vi "CANOpen Enter Frame Information.vi"(5 "Type":T3=enum."TPDO", 7 "Edit?":bool, 8 "error in (no error)":errorcluster, 9 "PDO Channel":u8(ring) items=["PDO 1", "PDO 2", "PDO 3", "PDO 4"], 10 "Parameters":T5[](array[typedef]) {"Bit Offset" max=8 step=1; "Byte Offset" max=8 step=1}, 11 "Node Ptr":u64 format="%.0x") -> (0 "error out":errorcluster, 1 "Cancelled?":bool, 2 "PDO Settings":T4={"Parameters"=[], "PDO Channel"=1, "Start Index"=1, "Length"=0} {"PDO Channel" items=["PDO 1", "PDO 2", "PDO 3", "PDO 4"]; "Parameters"."Bit Offset" max=8 step=1; "Parameters"."Byte Offset" max=8 step=1}, 3 "Item Ref out":T8 format="%.0x")   [LabVIEW 2021, in "CANOpen Addon System Explorer.lvlib"]
uses:
  CANOpen Addon System Explorer.lvlib
  <vilib>/NI VeriStand/Custom Device API/Custom Device Item Ref.ctl
  Shared/CANOpen_PDO Parameter Settings.ctl
  Shared/CANOpen_PDO Data Type.ctl
  CANopen Byte Order.ctl
  Shared/CANOpen_PDO Settings.ctl
  CANOpen_PDO Type.ctl
  Import.ctl
  Export.ctl
  <vilib>/NI VeriStand/Custom Device API/Custom Device API.lvlib
  Shared/CANOpen Addon Shared.lvlib
panel:
  in  "Import":T1
  in  "Export":T2
  in  "Cancel Button":bool
  in  "OK Button":bool
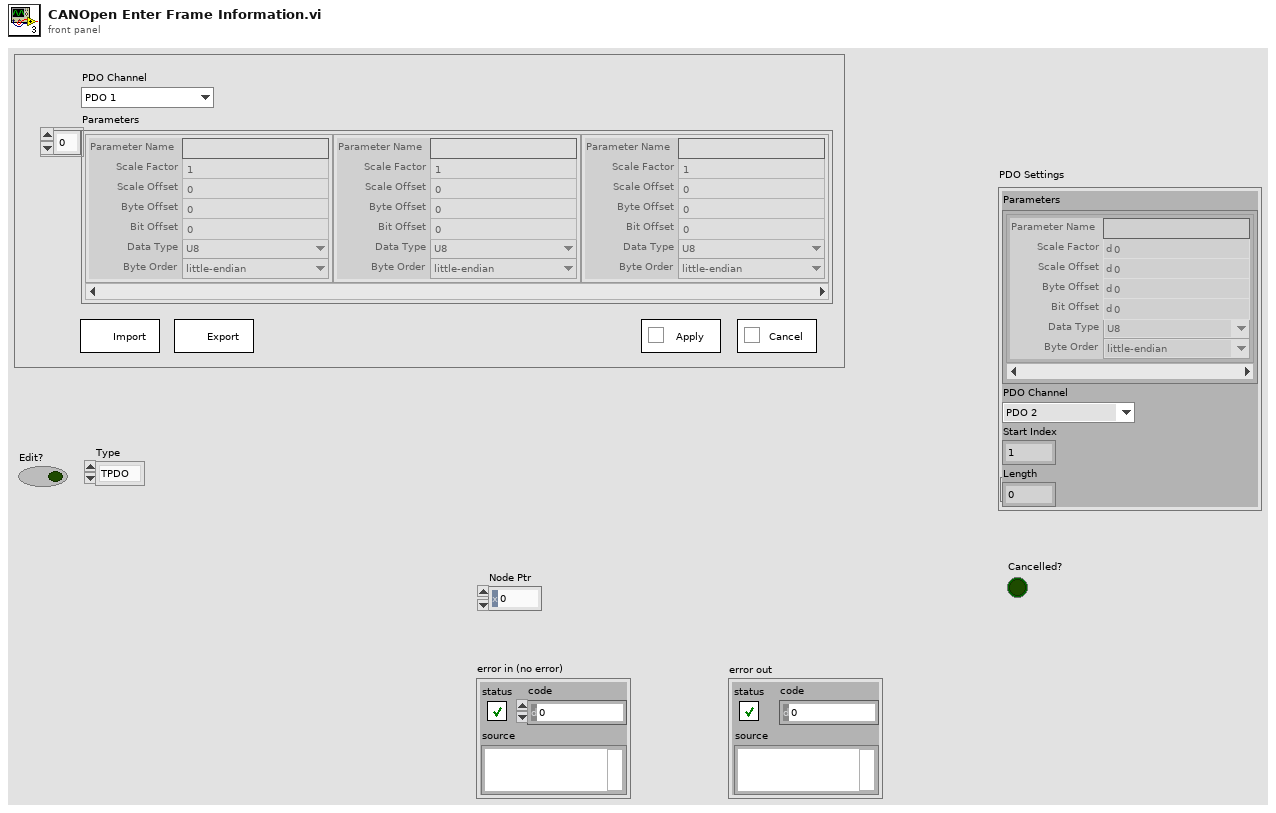
[diagram p1: front panel]
types:
  T1 = typedef "CANOpen Addon System Explorer.lvlib/Import.ctl" = bool
  T2 = typedef "CANOpen Addon System Explorer.lvlib/Export.ctl" = bool
  T3 = typedef "CANOpen Addon System Explorer.lvlib/CANOpen_PDO Type.ctl" = enum16{"RPDO", "TPDO"}
  T4 = typedef "CANOpen Addon Shared.lvlib/CANOpen_PDO Settings.ctl" = cluster{"Parameters":T5[], "PDO Channel":u8, "Start Index":u32, "Length":u32}
  T5 = typedef "CANOpen Addon Shared.lvlib/CANOpen_PDO Parameter Settings.ctl" = cluster{"Parameter Name":string, "Scale Factor":dbl, "Scale Offset":dbl, "Byte Offset":u8, "Bit Offset":u8, "Data Type":T6, "Byte Order":T7}
  T6 = typedef "CANOpen Addon Shared.lvlib/CANOpen_PDO Data Type.ctl" = enum16{"U8", "U16", "U32", "I8", "I16", "I32", "Single", "Double", "Boolean"}
  T7 = typedef "CANOpen Addon System Explorer.lvlib/CANopen Byte Order.ctl" = enum16{"big-endian network order", "little-endian"}
  T8 = typedef "Custom Device API.lvlib/Custom Device Item Ref.ctl" = u64
  T9 = typedef "Custom Device API.lvlib/Custom Device Item Info.ctl" = cluster{"Name":string, "Is Channel":bool, "GUID":string, "Is Waveform":bool}
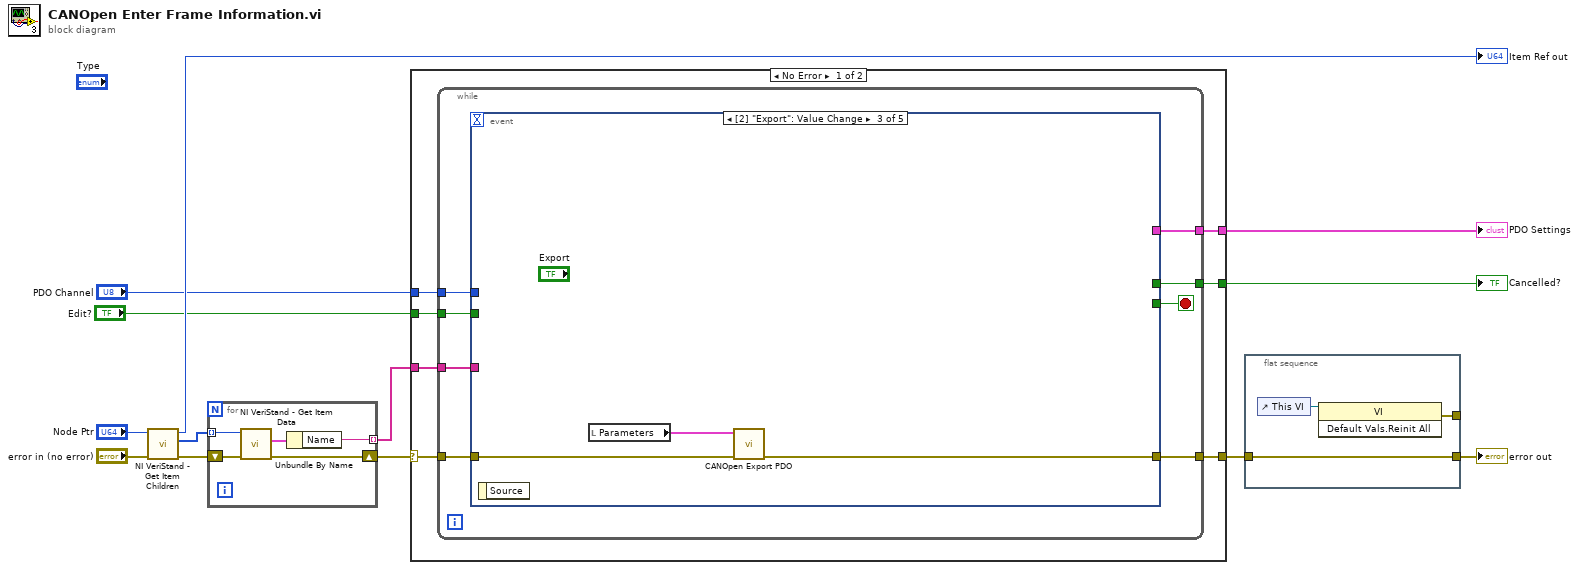
[diagram p0: block diagram]
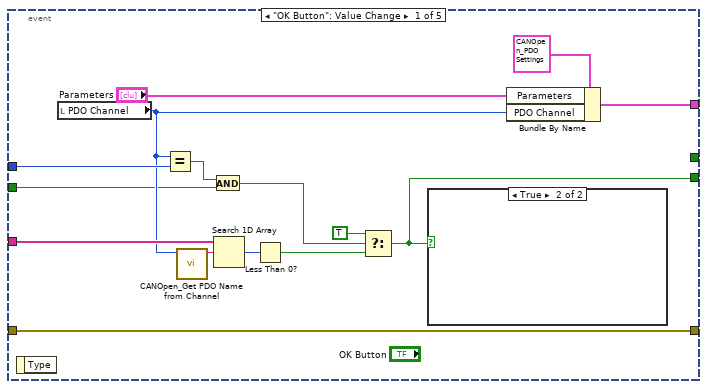
[diagram p2: hidden frame]
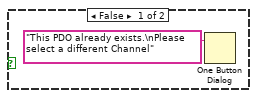
[diagram p3: hidden frame]
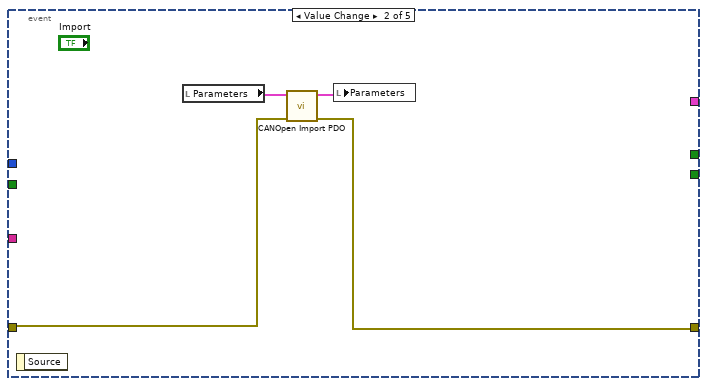
[diagram p4: hidden frame]
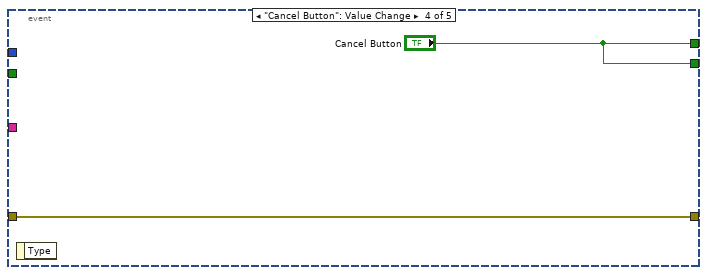
[diagram p5: hidden frame]
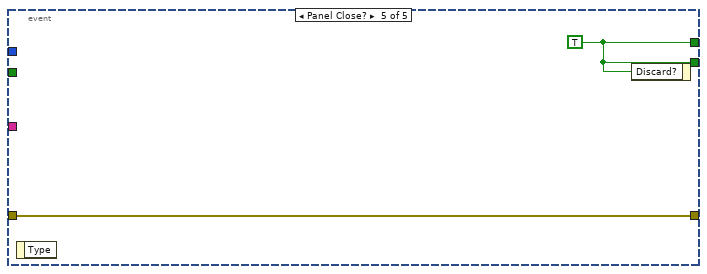
[diagram p6: hidden frame]
diagram:
  n1 = call <vilib>:"NI VeriStand - Get Item Children.vi"("error in (no error)"="error in (no error)", "Item Ref in"="Node Ptr") -> ("error out"=w12:errorcluster, "Child Refs"=w10:T8[], "Item Ref out"=→"Item Ref out":T8)  [unwired: 6 in, 1 out]
  n2 = for {
    tunnel: w10 -> [w17] mode=indexing
    tunnel: [w14] -> w9 mode=indexing
    shift-right: [w15] -> w11
    shift-left: w12 -> [w16]
    n3 = call <vilib>:"NI VeriStand - Get Item Data.vi"("error in (no error)"=w16, "Item Ref in"=w17) -> ("error out"=w15:errorcluster, "Item Info"=w18:T9)  [unwired: 6 in, 2 out]
    n4 = Unbundle By Name(w18) -> ("Name"=w14:string)
  }
  n5 = case shown="No Error" w11 {
    selector: w11 -> [w22 w61]
    tunnel: [w25 w61] -> w3
    tunnel: w9 -> [w24 _]
    tunnel: [w23 _] -> w13
    tunnel: [w21 _] -> w5
    tunnel: "PDO Channel" -> [w20 _]
    tunnel: "Edit?" -> [w19 _]
    frame No Error {
      n6 = while {
        tunnel: [w33] -> w25
        tunnel: w22 -> [w32]
        tunnel: w24 -> [w31]
        tunnel: [w29] -> w23
        tunnel: [w28] -> w21
        tunnel: w20 -> [w27]
        tunnel: w19 -> [w26]
        stop <- w30 stop-if-true
        n7 = event shown="[2] \"Export\": Value Change" {
          selector: _ -> [_ _ _ _ _]
          dyn-events: _ -> [_ _ _ _ _]
          timeout: _ -> [_ _ _ _ _]
          tunnel: [w46 w50 w55 w58 w60] -> w33
          tunnel: w32 -> [w46 w51 w56 w58 w60]
          tunnel: w31 -> [w48 _ _ _ _]
          tunnel: [w34 _ _ "Cancel Button" w59] -> w30
          tunnel: [_ _ _ "Cancel Button" w59] -> w29
          tunnel: [w44 _ _ _ _] -> w28
          tunnel: w27 -> [w41 _ _ _ _]
          tunnel: w26 -> [w38 _ _ _ _]
          event "OK Button": Value Change {
            n8 = event-data() -> ()  [unwired: 1 in, 1 out]
            n9 = local read "PDO Channel"() -> (w40:u8)
            n10 = Equal?(x=w40, y=w41) -> (x = y?=w39:bool)
            n11 = call "CANOpen_Get PDO Name from Channel.vi"("PDO Channel"=w40) -> ("PDO Channel Name"=w43:string)  [unwired: 10 in]
            n12 = And(x=w39, y=w38) -> (x .and. y?=w37:bool)
            n13 = Search 1D Array(1D array=w48, element=w43) -> (index of element=w47:i32)  [unwired: 1 in]
            n14 = Less Than 0?(x=w47) -> (x < 0?=w35:bool)
            n15 = Select(t=TRUE, s=w37, f=w35) -> (s? t:f=w34:bool)
            n16 = case shown="True" w34 {
              frame False {
                n17 = One Button Dialog(message="This PDO already exists.\nPlease select a different Channel") -> ()  [unwired: 1 in, 1 out]
              }
              frame True {
              }
            }
            n18 = Bundle By Name(cluster=T4 {"Parameters"=[{"Parameter Name"="", "Scale Factor"=0.0, "Scale Offset"=0.0, "Byte Offset"=0, "Bit Offset"=0, "Data Type"=enum."U8", "Byte Order"=enum."little-endian"}], "PDO Channel"=0, "Start Index"=1, "Length"=0} ("PDO Settings"), "Parameters"="Parameters", "PDO Channel"=w40) -> (w44:T4)
          }
          event Value Change {
            n19 = event-data() -> ()  [unwired: 1 in, 1 out]
            n20 = local read "Parameters"() -> (w53:T5[])
            n21 = call "CANOpen Import PDO.vi"("error in (no error)"=w51, "PDO in"=w53) -> ("error out"=w50:errorcluster, "PDO out"=w52:T5[])  [unwired: 8 in]
            n22 = local write "Parameters"(w52) -> ()
          }
          event Value Change {
            n23 = event-data() -> ()  [unwired: 1 in, 1 out]
            n24 = local read "Parameters"() -> (w54:T5[])
            n25 = call "CANOpen Export PDO.vi"("error in (no error)"=w56, "PDO in"=w54) -> ("error out"=w55:errorcluster)  [unwired: 9 in]
          }
          event "Cancel Button": Value Change {
            n26 = event-data() -> ()  [unwired: 1 in, 1 out]
          }
          event Panel Close? {
            w59 = TRUE ("Cancel Button")
            n27 = event-data() -> ()  [unwired: 1 in, 1 out]
            n28 = event-data("Discard?"=w59) -> ()  [unwired: 1 in, 1 out]
          }
        }
      }
    }
    frame Error {
    }
  }
  "Cancelled?" <- w13
  "PDO Settings" <- w5
  n29 = flat-sequence {
    tunnel: [w64] -> w4
    tunnel: w3 -> [w64]
    tunnel: [w62] -> _
    frame #0 {
      n30 = control-ref of="This VI"() -> (w63:refnum<vi>)
      n31 = invoke class="VI" method="Default Vals.Reinit All"(reference=w63) -> (error out=w62:errorcluster)  [unwired: 2 in, 2 out]
    }
  }
  "error out" <- w4
